vi "arbitrarySessionLogging.vi"(0 "file path in":path, 1 "Column Names":string[](array[string]), 2 "Log Values":dbl[](array[numeric]), 5 "Logging?":bool, 9 "Log on previous loop":bool, 11 "error in (no error)":errorcluster, 12 "Logging File Name":string) -> (4 "file path out":path, 10 "Log for next loop":bool, 15 "error out":errorcluster)   [LabVIEW 2025]
doc: "Creates .csv file and continuously updates file at \neach iteration of main program cycle. Date and \ntime are automatically appended to user selected\n\"Logging File Name\" input string and file is saved\nto file path \"...\\Labview_Logging\\...\" in project \nfolder. Logging is arbitrarily reinitialised with a \nunique path at each instance of a rising edge of\n\"Logging?\" input variable.\nNOTE: Subvi can handle log lengths of arbitrary \nsize BUT \"Column Names\" and \"Log Values\" \nsubvi inputs must be same dimension.\n\nINPUTS:\n 1. File path input -- should enter from shift \n register with prev. execution of subvi as feed.\n 2. Logging? -- Set true to initialise and maintain\n log file.\n 3. Log on previous loop -- tracking for logging\n rising edge reinitialisation. \n should enter from shift \n register with prev. \"Log for next loop\" subvi \n output as feed.\n 4. error in\n 4. Column Names -- Header column titles for\n subvi generated .csv file.\n 5. Log values -- values to enter into row n of \n generated .csv file.\n 6. Logging File Name -- user selected log file \n name.\n\nOUTPUTS:\n 1. file path out -- should exit into shift register\n passed into \"File path input\" of subvi at next \n program cycle.\n 2. Log for next loop -- tracking for logging\n rising edge reinitialisation. \n should exit into shift register passed into \"Log\n on previous loop\" of subvi at next program\n cycle."
uses:
  <vilib>/Utility/file.llb/Write Delimited Spreadsheet (string).vi
  <vilib>/Utility/file.llb/Write Delimited Spreadsheet (DBL).vi
panel:
  # "Arbitrary Logging\n\nCreates .csv file and continuously updates file at \neach iteration of main program cycle. Date and \ntime are automatically appended to user selected\n\"Logging File Name\" input string and file is saved\nto file path \"...\\Labview_Logging\\...\" in project \nfolder. Logging is arbitrarily reinitialised with a \nunique path at each instance of a rising edge of\n\"Logging?\" input variable.\nNOTE: Subvi can handle log lengths of arbitrary \nsize BUT \"Column Names\" and \"Log Values\" \nsubvi inputs must be same dimension.\n\nINPUTS:\n  1. File path input -- should enter from shift \n      register with prev. execution of subvi as feed.\n  2. Logging? -- Set true to initialise and maintain\n      log file.\n  3. Log on previous loop -- tracking for logging\n      rising edge reinitialisation. \n      should enter from shift \n      register with prev. \"Log for next loop\" subvi \n      output as feed.\n  4. error in\n  4. Column Names -- Header column titles for\n      subvi generated .csv file.\n  5. Log values -- values to enter into row n of \n      generated .csv file.\n  6. Logging File Name -- user selected log file \n      name.\n\nOUTPUTS:\n   1. file path out -- should exit into shift register\n    passed into \"File path input\" of subvi at next \n    program cycle.\n   2. Log for next loop -- tracking for logging\n      rising edge reinitialisation. \n      should exit into shift register passed into \"Log\n      on previous loop\" of subvi at next program\n      cycle."
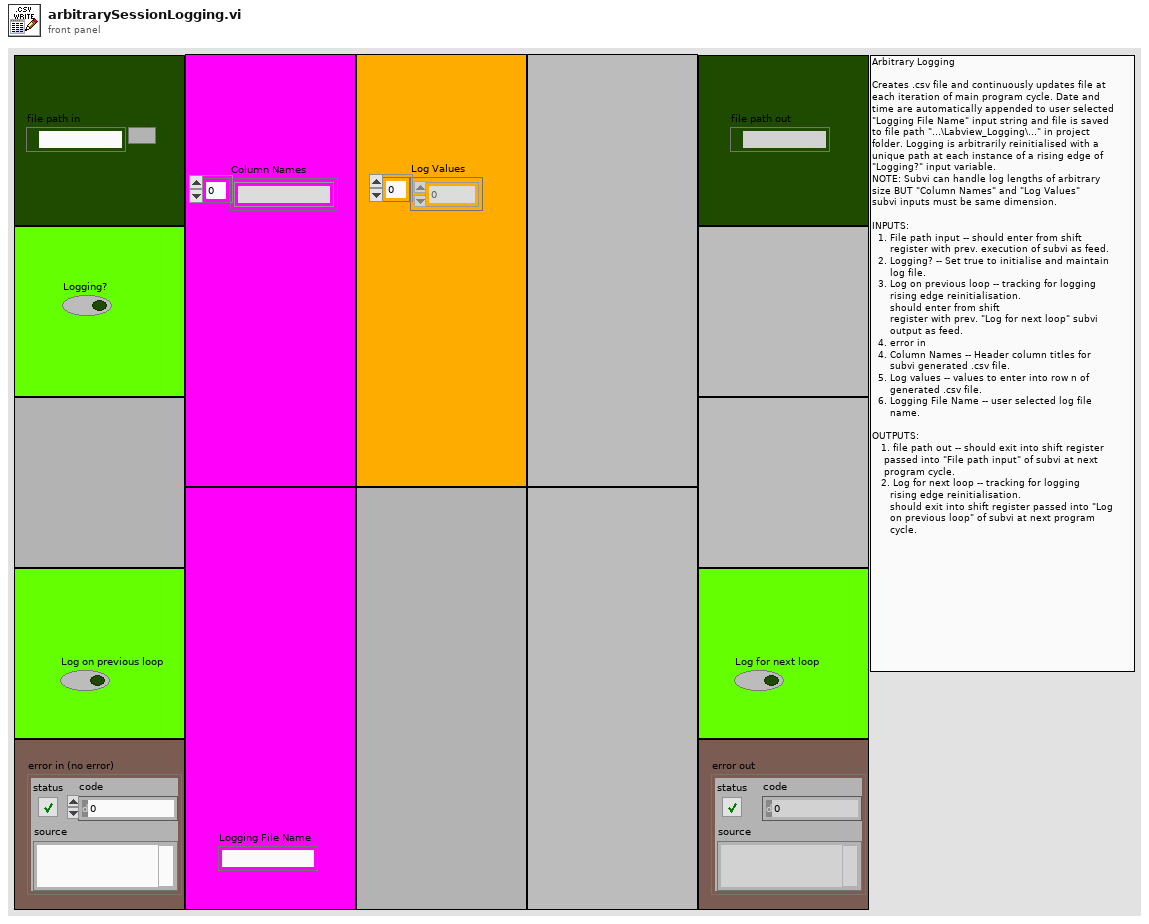
[diagram p1: front panel]
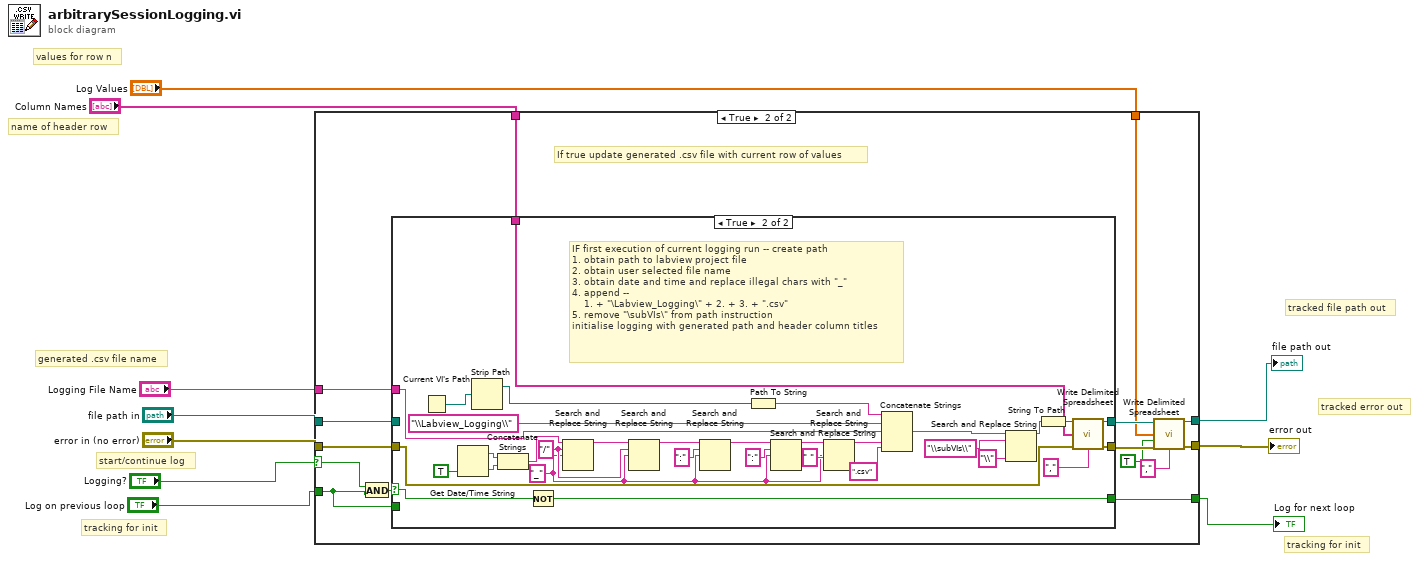
[diagram p0: block diagram]
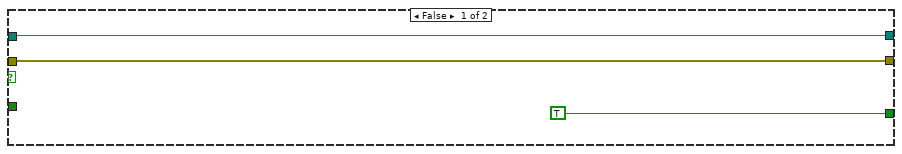
[diagram p2: hidden frame]
diagram:
  # "start/continue log"
  # "tracking for init"
  # "tracked error out"
  # "tracked file path out"
  # "tracking for init"
  # "generated .csv file name"
  # "values for row n"
  # "name of header row"
  n1 = case shown="True" "Logging?" {
    selector: "Logging?" -> [_ w16]
    tunnel: "Column Names" -> [_ w26]
    tunnel: "Log Values" -> [_ w25]
    tunnel: [w13 w23] -> w3
    tunnel: [w12 w22] -> w4
    tunnel: "file path in" -> [w13 w21]
    tunnel: "error in (no error)" -> [w12 w20]
    tunnel: "Logging File Name" -> [_ w19]
    tunnel: "Log on previous loop" -> [_ w15]
    tunnel: [TRUE w17] -> w9
    frame False {
    }
    frame True {
      # "If true update generated .csv file with current row of values"
      n2 = And(x=w16, y=w15) -> (x .and. y?=w18:bool)
      n3 = case shown="True" w18 {
        selector: w18 -> [_ w55]
        tunnel: [w29 w62] -> w28
        tunnel: [w30 w61] -> w27
        tunnel: w26 -> [_ w60]
        tunnel: w21 -> [w29 _]
        tunnel: w20 -> [w30 w59]
        tunnel: w19 -> [_ w56]
        tunnel: [w31 w54] -> w17
        tunnel: w15 -> [w31 _]
        frame False {
          # "if not initialising pass path and error lines"
        }
        frame True {
          w36 = "_" ("search string")
          w44 = "/" ("search string")
          # "IF first execution of current logging run -- create path\n1. obtain path to labview project file\n2. obtain user selected file name\n3. obtain date and time and replace illegal chars with \"_\"\n4. append --\n    1. + \"\\Labview_Logging\\\" + 2. + 3. + \".csv\"\n5. remove \"\\subVIs\\\" from path instruction\ninitialise logging with generated path and header column titles"
          n4 = Current VI's Path() -> (path=w52:path)
          n5 = Get Date/Time String(want seconds? (F)=TRUE) -> (date string=w47:string, time string=w48:string)  [unwired: 2 in]
          n6 = Strip Path(path=w52) -> (stripped path=w51:path)  [unwired: 1 out]
          n7 = Concatenate Strings(w47, w48) -> (w46:string)
          n8 = Not(x=w55) -> (.not. x?=w54:bool)
          n9 = Search and Replace String(input string=w46, search string=w44, replace string=w36) -> (result string=w45:string)  [unwired: 5 in, 3 out]
          n10 = Search and Replace String(input string=w45, search string=w44, replace string=w36) -> (result string=w43:string)  [unwired: 5 in, 3 out]
          n11 = Search and Replace String(input string=w43, search string=":", replace string=w36) -> (result string=w38:string)  [unwired: 5 in, 3 out]
          n12 = Path To String(path=w51) -> (string=w58:string)
          n13 = Search and Replace String(input string=w38, search string=":", replace string=w36) -> (result string=w37:string)  [unwired: 5 in, 3 out]
          n14 = Search and Replace String(input string=w37, search string=" ", replace string=w36) -> (result string=w41:string)  [unwired: 5 in, 3 out]
          n15 = Concatenate Strings(w58, "\\Labview_Logging\\" ("delimiter (\\t)"), w56, w41, ".csv" ("delimiter (\\t)")) -> (w34:string)
          n16 = Search and Replace String(input string=w34, search string="\\subVIs\\", replace string="\\" ("replace string (\"\")")) -> (result string=w35:string)  [unwired: 5 in, 3 out]
          n17 = String To Path(string=w35) -> (path=w53:path)
          n18 = call-poly <vilib>:"Write Delimited Spreadsheet.vi"("file path (dialog if empty)"=w53, "1D data"=w60, "error in (no error)"=w59, "delimiter (\\t)"="," ("delimiter (\\t)")) -> ("new file path (Not A Path if cancelled)"=w62:path, "error out"=w61:errorcluster)  [unwired: 10 in]
        }
      }
      n19 = call-poly <vilib>:"Write Delimited Spreadsheet.vi"("file path (dialog if empty)"=w28, "1D data"=w25, "append to file? (new file:F)"=TRUE, "error in (no error)"=w27, "delimiter (\\t)"="," ("delimiter (\\t)")) -> ("new file path (Not A Path if cancelled)"=w23:path, "error out"=w22:errorcluster)  [unwired: 9 in]
    }
  }
  "Log for next loop" <- w9
  "error out" <- w4
  "file path out" <- w3
